vi "Master_NavigationLoop.vi"(8 "error in (no error)":errorcluster) -> (0 "error out":errorcluster)   [LabVIEW 2018]
uses:
  Type_Def/TypeDef_LoopPeriod.ctl
  Type_Def/Master_DataControl.ctl
  Type_Def/TypeDef_cRIODatas.ctl
  Type_Def/Type_Def IMUDatas.ctl
  Type_Def/TypeDef_BMSDatas.ctl
  Type_Def/TypeDef_BMSStatuss.ctl
  Type_Def/TypeDef FixedMotorData.ctl
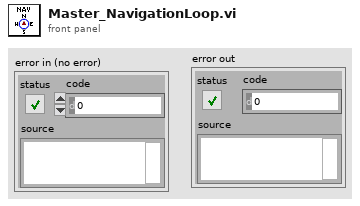
[diagram p1: front panel]
types:
  T1 = typedef "TypeDef_LoopPeriod.ctl" = cluster{"Control Period":i64, "DAQ Period":u32, "IMU Period":u32, "CAN Period":i64, "Nav Period":u32}
  T2 = typedef "Master_DataControl.ctl" = cluster{"cRIO Data":T3, "IMU Data":T4, "BMS Data":T5, "Motor Data":T7}
  T3 = typedef "TypeDef_cRIODatas.ctl" = cluster{"HallEffect Right (cm)":dbl, "HallEffect Left (cm)":dbl, "Optical Sensor 1 (V)":dbl, "Optical Sensor 2 (V)":dbl, "24V Voltage  (V)":dbl, "24V Current (A)":dbl, "Contactor H1 Continuity":dbl, "Contactor L1 Continuity ":dbl, "Contactor H2 Continuity":dbl, "Contactor L2 Continuity ":dbl, "Brake PT(psig)":dbl, "Pump PT (psig)":dbl, "24V Temp   (C)":dbl, "Tank PT(psig) ":dbl, "ABS Pressure 1 (psig)":dbl, "ABS Pressure 2 (psig) ":dbl, "Displacement (ft)":dbl, "Velocity (ft/s)":dbl, "Time (ms)":dbl, "PV 1 Temp":dbl, "PV2 Temp":dbl}
  T4 = typedef "Type_Def IMUDatas.ctl" = cluster{"y acceleration (g)":dbl, "Pressure (psia)":dbl, "Temperature (F)":dbl}
  T5 = typedef "TypeDef_BMSDatas.ctl" = cluster{"Pack 1 Max Cell\n Voltage (V)":dbl, "Pack 1 Max Cell\n ID ":dbl, "Pack 1 Min Cell \nVoltage (V)":dbl, "Pack 1 Min Cell \nID ":dbl, "Pack 1 State of Charge  (%)":dbl, "Pack 1 Average Voltage1 (V)":dbl, "Pack 1Voltage Delta (V)":dbl, "Pack 1 Current (A)":dbl, "Pack 1 Voltage (V)":dbl, "Pack 1 Max Resistance (Ohm)":dbl, "Pack 1Min Resistance (Ohm)":dbl, "Pack 1Average Resistance (Ohm)":dbl, "Pack 1Delta Resistance (Ohm)":dbl, "Pack 1 Highest Temperature(F)":dbl, "BmsStatus1":T6, "Pack 2 Max Cell\n Voltage (V) ":dbl, "Pack 2 Max Cell\n ID  ":dbl, "Pack 2 Min Cell \nVoltage (V) ":dbl, "Pack 2 Min Cell \nID  ":dbl, "Pack 2 Average Voltage1 (V)":dbl, "Pack 2 Voltage Delta (V) ":dbl, "Pack 2 Current (A)":dbl, "Pack 2 Voltage (V) ":dbl, "Pack 2 State of Charge  (%) ":dbl, "Pack 2 Max Resistance (Ohm) ":dbl, "Pack 2 Min Resistance (Ohm)":dbl, "Pack 2 Average Resistance (Ohm)":dbl, "Pack 2 Delta Resistance (Ohm) ":dbl, "Pack 2 Highest Temperature(F) ":dbl, "BmsStatus 2":T6}
  T6 = typedef "TypeDef_BMSStatuss.ctl" = cluster{"isFault":bool, "isolationMonitoring":bool}
  T7 = typedef "TypeDef FixedMotorData.ctl" = cluster{" Velocity (RPM)":dbl, " MotorTemp(C)":dbl, " ControlTemp(C)":dbl, " DcLinkVolt(V)":dbl, " ErrorCode":dbl, "IsAlive":bool, "motorStatus":cluster{"isReady":bool, "isOn":bool, "isOperEn":bool, "isFault":bool, "isVoltEn":bool, "targetReached":bool, "isWarning":bool}, "motorControllerState":u16}
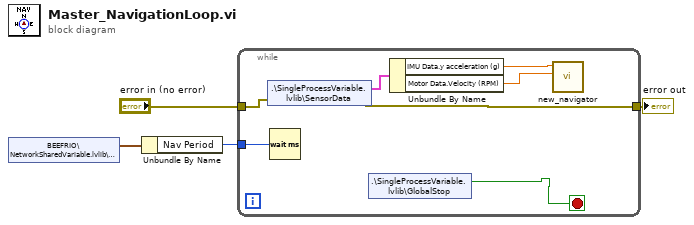
[diagram p0: block diagram]
diagram:
  n1 = shared-variable "BEEFRIO\\NetworkSharedVariable.lvlib\\LoopPeriods"() -> (w3:T1)  [unwired: 1 in, 1 out]
  n2 = Unbundle By Name(w3) -> ("Nav Period"=w2:u32)
  n3 = while {
    tunnel: "error in (no error)" -> [w10]
    tunnel: w2 -> [w9]
    tunnel: [w8] -> w1
    stop <- w7 stop-if-true
    n4 = shared-variable ".\\SingleProcessVariable.lvlib\\SensorData"(error in=w10) -> (w11:T2, error out=w8:errorcluster)
    n5 = Wait (ms)(milliseconds to wait=w9) -> ()  [unwired: 1 out]
    n6 = shared-variable ".\\SingleProcessVariable.lvlib\\GlobalStop"() -> (w7:bool)  [unwired: 1 in, 1 out]
    n7 = Unbundle By Name(w11) -> ("IMU Data.y acceleration (g)"=w6:dbl, "Motor Data.Velocity (RPM)"=w5:dbl)
    n8 = call "new_navigator.vi"("velocity from motor Controllor (m/s)"=w5, "y acceleration (g)"=w6) -> ()  [unwired: 10 in]
  }
  "error out" <- w1
